vi "Configure Measurement.vi"(0 "VISA resource name":refnum<visa-resource-name>, 1 "Scan List (Empty)":string, 5 "Function (0: DC Voltage)":u16(ring) items=["DC Voltage", "AC Voltage", "DC Current", "AC Current", "Resistance", "Four-Wire Resistance", "Temperature", "Frequency", "Period", "Continuity"], 7 "Resolution (3: 6.5 Digits)":u16(ring)=3 items=["3.5", "4.5", "5.5", "6.5"], 9 "Enable Auto Range (True)":bool=TRUE, 11 "error in (no error)":errorcluster, 12 "Manual Range (10)":dbl=10.0) -> (4 "VISA resource name out":refnum<visa-resource-name>, 15 "error out":errorcluster)   [LabVIEW 2015, in "Keithley 27XX.lvlib"]
doc: "This VI sets the measurement function as well as a Range and Resolution for that function when allowed by the instrument.\n\nNote: \n(1) Temperature: Does not allow configuration of Range\nFrequency: Does not allow configuration of Range\nPeriod: Does not allow configuration of Range\nContinuity: Does not allow configuration of Range or Resolution\n\n(2) Resolution is sometimes refered to as Digits of precision. \n\n(3) Error -1073999873 is generated if the Scan List control does not correctly correspond with the Front/Rear Input Switch."
uses:
  Keithley 27XX.lvlib
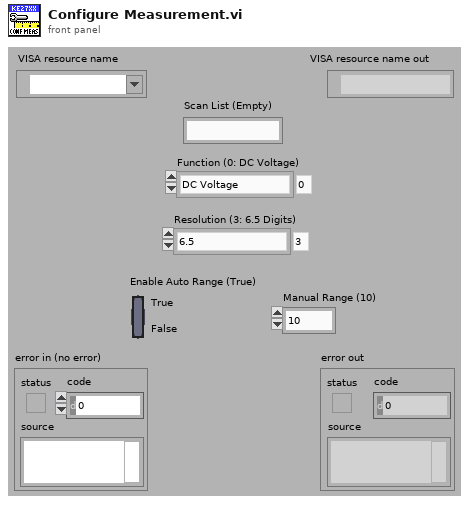
[diagram p1: front panel]
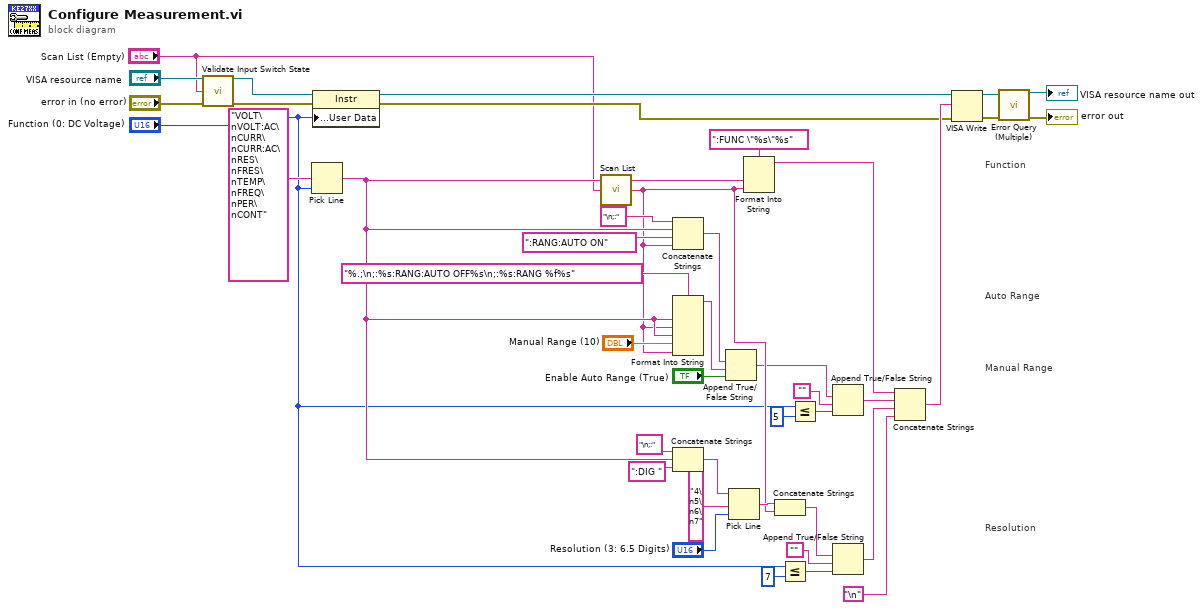
[diagram p0: block diagram]
diagram:
  # "Resolution"
  # "Manual Range"
  # "Auto Range"
  # "Function"
  n1 = call "Validate Input Switch State.vi"("VISA resource name"="VISA resource name", "Scan List (Empty: front panel)"="Scan List (Empty)", "error in (no error)"="error in (no error)") -> ("VISA resource name out"=w3:refnum<visa-resource-name>, "error out"=w2:errorcluster)  [unwired: 10 in, 1 out]
  n2 = Pick Line(multi-line string="VOLT\nVOLT:AC\nCURR\nCURR:AC\nRES\nFRES\nTEMP\nFREQ\nPER\nCONT", line index="Function (0: DC Voltage)") -> (output string=w26:string)  [unwired: 1 in]
  n3 = property on="Property Node" class="Instr"(reference=w3, error in=w2, "General Settings:User Data"="Function (0: DC Voltage)") -> (reference out=w30:refnum<visa-resource-name>, error out=w29:errorcluster)
  n4 = call "Scan List.vi"("Scan List (Empty)"="Scan List (Empty)") -> ("Scan List Out"=w12:string)  [unwired: 14 in]
  n5 = Concatenate Strings("\n;:" ("string"), w26, ":RANG:AUTO ON", w12) -> (w32:string)
  n6 = Format Into String(format string="%.;\n;:%s:RANG:AUTO OFF%s\n;:%s:RANG %f%s" ("string"), w26, w12, w26, "Manual Range (10)", w12) -> (resulting string=w33:string)  [unwired: 2 in, 1 out]
  n7 = Concatenate Strings("\n;:" ("string"), w26, ":DIG " ("string")) -> (w38:string)
  n8 = Append True/False String(1:"Enable Auto Range (True)", 2:w33, 3:w32) -> (0:w7:string)  [unwired: 1 in]
  n9 = Pick Line(string ("")=w38, multi-line string="4\n5\n6\n7", line index="Resolution (3: 6.5 Digits)") -> (output string=w13:string)
  n10 = Format Into String(format string=":FUNC \"%s\"%s", w26, w12) -> (resulting string=w28:string)  [unwired: 2 in, 1 out]
  n11 = Concatenate Strings(w13, w12) -> (w11:string)
  n12 = Less Or Equal?(x="Function (0: DC Voltage)", y=7) -> (x <= y?=w17:bool)
  n13 = Less Or Equal?(x="Function (0: DC Voltage)", y=5) -> (x <= y?=w18:bool)
  n14 = Append True/False String(1:w18, 2:"", 3:w7) -> (0:w10:string)  [unwired: 1 in]
  n15 = Append True/False String(1:w17, 2:"", 3:w11) -> (0:w14:string)  [unwired: 1 in]
  n16 = Concatenate Strings(w28, w10, w14, "\n") -> (w41:string)
  n17 = VISA Write(VISA resource name=w30, write buffer=w41, error in (no error)=w29) -> (VISA resource name out=w24:refnum<visa-resource-name>, error out=w23:errorcluster)  [unwired: 1 out]
  n18 = call "Error Query (Multiple).vi"("VISA resource name"=w24, "error in (no error)"=w23) -> ("VISA resource name out"=→"VISA resource name out":refnum<visa-resource-name>, "error out"=→"error out":errorcluster)  [unwired: 10 in, 2 out]
